vi "FeasaOpenCom.vi"(8 "error in (no error)":errorcluster, 11 "VISA resource name":refnum<visa-resource-name>="COM12") -> (0 "error out":errorcluster, 3 "VISA out":refnum<visa-resource-name>)   [LabVIEW 2025]
doc: "Open Comm port for Feasa LED Analyser.\n\nInput:\n- VISA in:\n Comm port in.\n\n- Error in:\n Error message in\n\nOutput:\n- VISA out:\n Comm port out\n\n- Error out:\n Error message out"
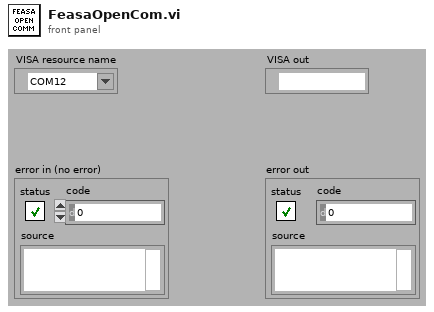
[diagram p1: front panel]
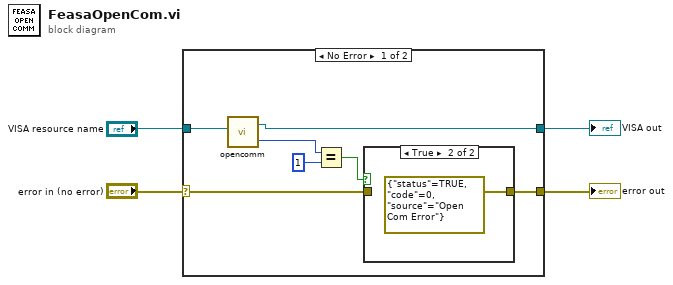
[diagram p0: block diagram]
diagram:
  n1 = case shown="No Error" "error in (no error)" {
    selector: "error in (no error)" -> [w6 w15]
    tunnel: "VISA resource name" -> [w11 w14]
    tunnel: [w5 w15] -> w2
    tunnel: [w10 w14] -> w1
    frame No Error {
      n2 = call "opencomm.vi"("VISA resource name"=w11) -> ("duplicate VISA resource name"=w10:refnum<visa-resource-name>, "Error"=w9:u16)
      n3 = Equal?(x=w9, y=u16 1) -> (x = y?=w7:bool)
      n4 = case shown="True" w7 {
        tunnel: [w12 errorcluster {"status"=TRUE, "code"=0, "source"="Open Com Error"} ("error constant")] -> w5
        tunnel: w6 -> [w12 _]
        frame False {
        }
        frame True {
        }
      }
    }
    frame Error {
    }
  }
  "error out" <- w2
  "VISA out" <- w1
